vi "S2C_PCIe1762H_Poly_TestBed.vi"() -> ()   [LabVIEW 2015]
uses:
  TypeDefs/S2C_PCIe1762H_Type_FootSwitch.ctl
  S2C_PCIe1762H_Poly_Initialize.vi
  S2C_PCIe1762H_Poly_FootSwitchWrite.vi
  S2C_PCIe1762H_Poly_FootSwitchRead.vi
  S2C_PCIe1762H_Poly_ResetAll.vi
panel:
  out "Error Out":errorcluster
  in  "Error In":errorcluster
  out "Response":T1
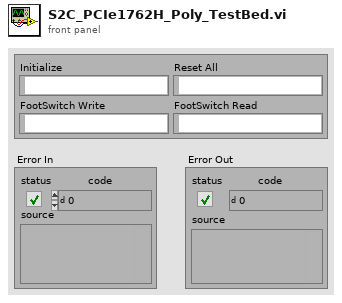
[diagram p1: front panel]
types:
  T1 = cluster{"Initialize":string, "FootSwitch Write":string, "FootSwitch Read":string, "Reset All":string}
  T2 = typedef "S2C_PCIe1762H_Type_FootSwitch.ctl" = u16
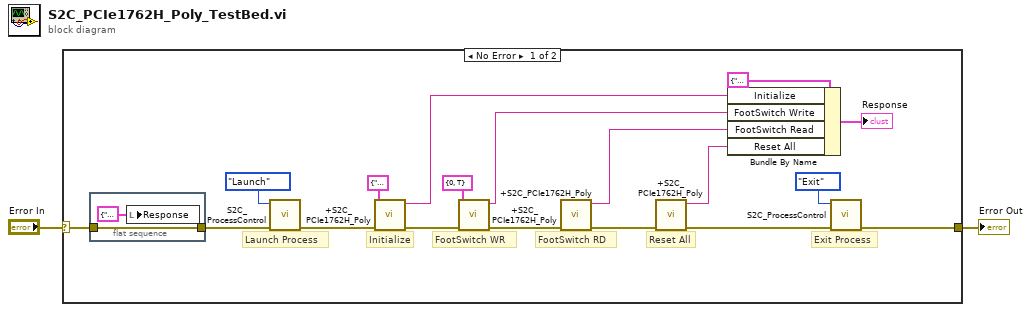
[diagram p0: block diagram]
diagram:
  n1 = case shown="No Error" "Error In" {
    selector: "Error In" -> [w17 w23]
    tunnel: [w18 w23] -> w1
    frame No Error {
      # "Reset All"
      # "Initialize"
      # "FootSwitch RD"
      # "FootSwitch WR"
      # "Exit Process"
      # "Launch Process"
      n2 = flat-sequence {
        tunnel: w17 -> [w22]
        tunnel: [w22] -> w16
        frame #0 {
          n3 = local write "Response"(T1 {"Initialize"="", "FootSwitch Write"="", "FootSwitch Read"="", "Reset All"=""} ("Response")) -> ()
        }
      }
      n4 = call "S2C_ProcessControl.vi"("Error In"=w16, "Action"=enum16{"Launch", "Exit"}."Launch") -> ("Error Out"=w11:errorcluster)  [unwired: 9 in]
      n5 = call-poly "+S2C_PCIe1762H_Poly.vi"("Error In"=w11, "Initialize"=cluster{"Device":string, "Module Index":u16} {"Device"="DemoDevice", "Module Index"=0}) -> ("Error Out"=w10:errorcluster, "Response"=w8:string)  [unwired: 8 in]
      n6 = call-poly "+S2C_PCIe1762H_Poly.vi"("Error In"=w10, "FootSwitch"=cluster{"FootSwitch":T2, "State":bool} {"FootSwitch"=0, "State"=TRUE}) -> ("Error Out"=w15:errorcluster, "Response"=w14:string)  [unwired: 8 in]
      n7 = call-poly "+S2C_PCIe1762H_Poly.vi"("Error In"=w15) -> ("Error Out"=w4:errorcluster, "Response"=w13:string)  [unwired: 9 in]
      n8 = call-poly "+S2C_PCIe1762H_Poly.vi"("Error In"=w4) -> ("Error Out"=w3:errorcluster, "Response"=w5:string)  [unwired: 9 in]
      n9 = Bundle By Name(cluster=T1 {"Initialize"="", "FootSwitch Write"="", "FootSwitch Read"="", "Reset All"=""} ("Response"), "Initialize"=w8, "FootSwitch Write"=w14, "FootSwitch Read"=w13, "Reset All"=w5) -> (→"Response":T1)
      n10 = call "S2C_ProcessControl.vi"("Error In"=w3, "Action"=enum16{"Launch", "Exit"}."Exit") -> ("Error Out"=w18:errorcluster)  [unwired: 9 in]
    }
    frame Error {
    }
  }
  "Error Out" <- w1
